vi "Create Auto-Populating Folder.vi"(0 "Project path":path, 5 "Plug-in name":string, 11 "error in (no error)":errorcluster) -> (4 "MeasurementCore reference":refnum<vi>, 6 "Folder reference":refnum<vi>, 8 "Project reference":refnum<vi>, 15 "error out":errorcluster)   [LabVIEW 2021, in "Multiple Migrator.lvlib"]
uses:
  Multiple Migrator.lvlib
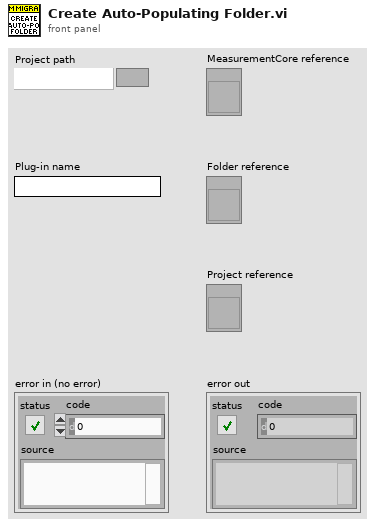
[diagram p1: front panel]
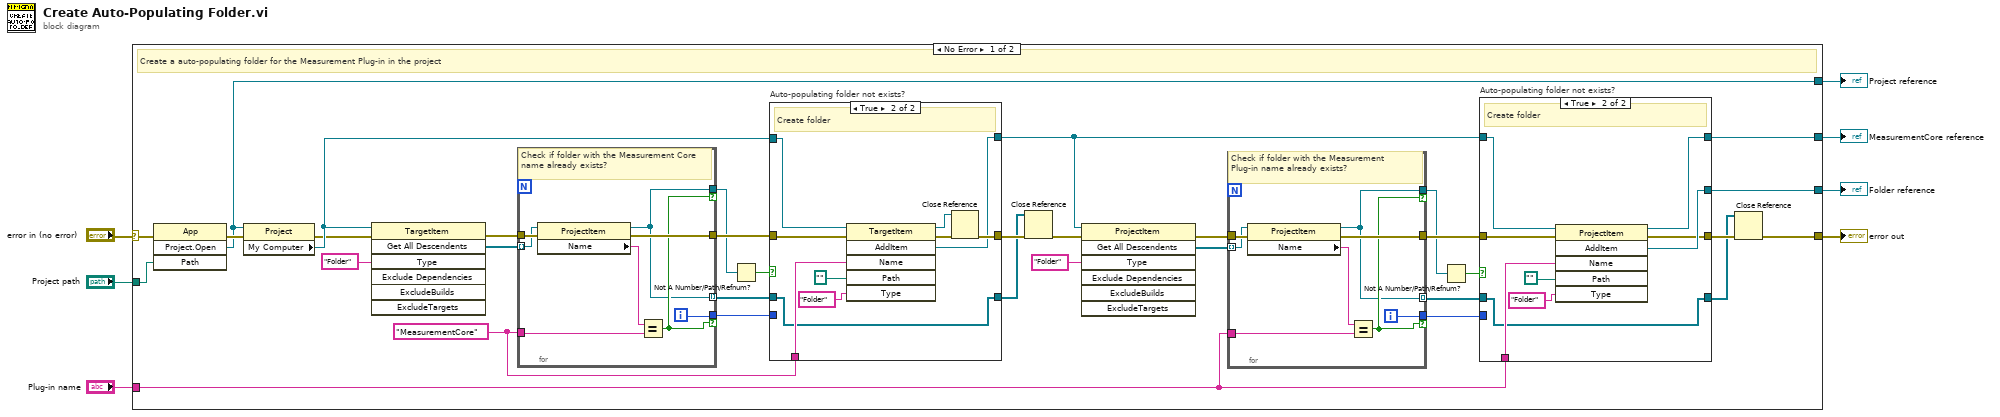
[diagram p0: block diagram]
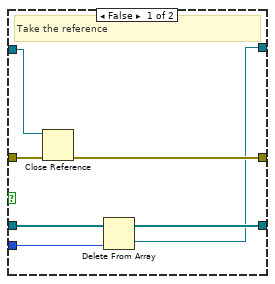
[diagram p2: hidden frame]
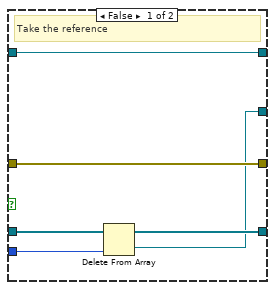
[diagram p3: hidden frame]
diagram:
  n1 = case shown="No Error" "error in (no error)" {
    selector: "error in (no error)" -> [w36 w89]
    tunnel: [w8 w89] -> w7
    tunnel: "Project path" -> [w30 _]
    tunnel: "Plug-in name" -> [w13 _]
    tunnel: [w11 _] -> w3
    tunnel: [w10 _] -> w2
    tunnel: [w9 _] -> w1
    frame No Error {
      w29 = "MeasurementCore"
      # "Create a auto-populating folder for the Measurement Plug-in in the project"
      n2 = invoke class="App" method="Project.Open"(error in=w36, "Path"=w30) -> (error out=w32:errorcluster, "Project:Open"=w9:refnum<vi>)  [unwired: 2 in, 2 out]
      n3 = property class="Project"(reference=w9, error in=w32) -> (error out=w33:errorcluster, "My Computer"=w38:refnum<vi>)  [unwired: 1 out]
      n4 = invoke class="TargetItem" method="Get All Descendents"(reference=w38, error in=w33, "Type"="Folder") -> (error out=w35:errorcluster, "All Descendents"=w31:refnum<vi>[])  [unwired: 4 in, 5 out]
      n5 = for {
        tunnel: w35 -> [w48]
        tunnel: w31 -> [w47] mode=indexing
        tunnel: [w41] -> w26 if=w42
        tunnel: [w45] -> w39
        tunnel: w29 -> [w44]
        tunnel: [w43] -> w28 if=w42
        tunnel: [w41] -> w27 mode=indexing
        i -> [w43]
        # "Check if folder with the Measurement Core name already exists?"
        n6 = property class="ProjectItem"(reference=w47, error in=w48) -> (reference out=w41:refnum<vi>, error out=w45:errorcluster, "Name"=w46:string)
        n7 = Equal?(x=w46, y=w44) -> (x = y?=w42:bool)
      }
      n8 = Not A Number/Path/Refnum?(number/path/refnum=w26) -> (NaN/Path/Refnum?=w37:bool)
      n9 = case "Auto-populating folder not exists?" shown="True" w37 {
        tunnel: w38 -> [w53 w65]
        tunnel: w39 -> [w55 w61]
        tunnel: [w54 w60] -> w40
        tunnel: w29 -> [_ w58]
        tunnel: [w49 w57] -> w12
        tunnel: w28 -> [w51 _]
        tunnel: w27 -> [w52 w56]
        tunnel: [w50 w56] -> w25
        frame False {
          # "Take the reference"
          n10 = Close Reference(reference=w53, error in (no error)=w55) -> (error out=w54:errorcluster)
          n11 = Delete From Array(array=w52, index=w51) -> (deleted portion=w49:refnum<vi>, array with subset deleted=w50:refnum<vi>[])  [unwired: 1 in]
        }
        frame True {
          # "Create folder"
          n12 = invoke class="TargetItem" method="AddItem"(reference=w65, error in=w61, "Name"=w58, "Path"=path "", "Type"="Folder") -> (reference out=w62:refnum<vi>, error out=w63:errorcluster, "AddItem"=w57:refnum<vi>)  [unwired: 1 in, 3 out]
          n13 = Close Reference(reference=w62, error in (no error)=w63) -> (error out=w60:errorcluster)
        }
      }
      n14 = Close Reference(reference=w25, error in (no error)=w40) -> (error out=w15:errorcluster)
      n15 = invoke class="ProjectItem" method="Get All Descendents"(reference=w12, error in=w15, "Type"="Folder") -> (error out=w21:errorcluster, "All Descendents"=w20:refnum<vi>[])  [unwired: 4 in, 5 out]
      n16 = for {
        tunnel: w21 -> [w73]
        tunnel: w20 -> [w72] mode=indexing
        tunnel: [w66] -> w17 if=w67
        tunnel: [w70] -> w23
        tunnel: w13 -> [w69]
        tunnel: [w68] -> w19 if=w67
        tunnel: [w66] -> w18 mode=indexing
        i -> [w68]
        # "Check if folder with the Measurement Plug-in name already exists?"
        n17 = property class="ProjectItem"(reference=w72, error in=w73) -> (reference out=w66:refnum<vi>, error out=w70:errorcluster, "Name"=w71:string)
        n18 = Equal?(x=w71, y=w69) -> (x = y?=w67:bool)
      }
      n19 = Not A Number/Path/Refnum?(number/path/refnum=w17) -> (NaN/Path/Refnum?=w22:bool)
      n20 = case "Auto-populating folder not exists?" shown="True" w22 {
        tunnel: w23 -> [w79 w87]
        tunnel: [w79 w81] -> w24
        tunnel: w13 -> [_ w85]
        tunnel: [w75 w84] -> w11
        tunnel: w19 -> [w77 _]
        tunnel: w18 -> [w78 w83]
        tunnel: [w76 w83] -> w16
        tunnel: w12 -> [w74 w82]
        tunnel: [w74 w80] -> w10
        frame False {
          # "Take the reference"
          n21 = Delete From Array(array=w78, index=w77) -> (deleted portion=w75:refnum<vi>, array with subset deleted=w76:refnum<vi>[])  [unwired: 1 in]
        }
        frame True {
          # "Create folder"
          n22 = invoke class="ProjectItem" method="AddItem"(reference=w82, error in=w87, "Name"=w85, "Path"=path "", "Type"="Folder") -> (reference out=w80:refnum<vi>, error out=w81:errorcluster, "AddItem"=w84:refnum<vi>)  [unwired: 1 in, 3 out]
        }
      }
      n23 = Close Reference(reference=w16, error in (no error)=w24) -> (error out=w8:errorcluster)
    }
    frame Error {
    }
  }
  "error out" <- w7
  "Folder reference" <- w3
  "MeasurementCore reference" <- w2
  "Project reference" <- w1
